vi "ShowRange.vi"(0 "File Info":T1={"FilePath"=path "/DATA/Labview Items", "Field (T)"=55.0, "Temperature (K)"=77.0, "X-Axis"=enum."nm", "Center nm"=55.0, "Current Grating Density"=enum."600", "CCD Parameters"={"Exposure Time (s)"=0.2, "Offset"=0.0, "BkgrdCrct"=FALSE, "Shutter"=FALSE, "Mode"=enum."Regular", "Repetition"=4, "dt or s"=0.0}, "Operation Mode"=enum."NML Data Acquisition", "Exp Index"=0, "Index_repetition"=0, "Index"=0, "Current Detector"=enum."CCD-1024x256"} {"CCD Parameters"."dt or s" format="%#.6f"; "CCD Parameters"."Repetition" min=1; "CCD Parameters"."Offset" format="%#.2f"; "CCD Parameters"."Exposure Time (s)" min=0.02 max=6000.0 format="%#.2f"; "Center nm" format="%.2f"; "Temperature (K)" format="%.2f"; "Field (T)" format="%.2f"}) -> ()   [LabVIEW 2020]
uses:
  Globals and TypeDefs/Type Definitions.llb/FileInfoParameter.ctt
  Globals and TypeDefs/Type Definitions.llb/Wavelength Unit.ctt
  Globals and TypeDefs/Type Definitions.llb/McPherson Grating Density.ctl
  Globals and TypeDefs/Type Definitions.llb/CCDParameter.ctt
  Globals and TypeDefs/Type Definitions.llb/OperationMode.ctt
  Globals and TypeDefs/Type Definitions.llb/ListOfDetectors.ctt
  X-Axis_Generator_x.vi
  X-Axis Converter.llb/X-Axis Converter.vi
panel:
  out "Old/Res/cm-1/500µ":dbl=118.16619973413901 caption="Old/Res/nm/10µ"
  out "Old/Res/cm-1/100µ":dbl=118.16619973413901 caption="Old/Res/nm/10µ" format="%.1f"
  out "New/Res/cm-1/500µ":dbl=25.810711007261716
  out "New/Res/cm-1/100µ":dbl=25.810711007261716 format="%.1f"
  out "Old/Res/cm-1/20µ":dbl=118.16619973413901 caption="Old/Res/nm/10µ" format="%.2f"
  out "New/Res/cm-1/20µ":dbl=25.810711007261716 format="%.2f"
  out "Old/Res/meV/500µ":dbl=118.16619973413901 caption="Old/Res/nm/10µ" format="%.1f"
  out "Old/Res/meV/100µ":dbl=118.16619973413901 caption="Old/Res/nm/10µ" format="%.2f"
  out "New/Res/meV/500µ":dbl=25.810711007261716 format="%.1f"
  out "New/Res/meV/100µ":dbl=25.810711007261716 format="%.2f"
  out "Old/Res/meV/20µ":dbl=118.16619973413901 caption="Old/Res/nm/10µ" format="%.3f"
  out "New/Res/meV/20µ":dbl=25.810711007261716 format="%.3f"
  out "Old/Res/nm/500µ":dbl=118.16619973413901 caption="Old/Res/nm/10µ" format="%.1f"
  out "Old/Res/nm/100µ":dbl=118.16619973413901 caption="Old/Res/nm/10µ" format="%.2f"
  out "New/Res/nm/500µ":dbl=25.810711007261716 format="%.1f"
  out "New/Res/nm/100µ":dbl=25.810711007261716 format="%.2f"
  out "Old/Res/nm/20µ":dbl=118.16619973413901 caption="Old/Res/nm/10µ" format="%.3f"
  out "New/Res/nm/20µ":dbl=25.810711007261716 format="%.3f"
  out "old cm-1 limit":dbl
  out "old meV limit":dbl
  out "old nm limit":dbl
  out "cm-1 limit":dbl
  out "meV limit":dbl
  out "nm limit":dbl
  out "Central WL output":dbl=619.92122 caption="Final Center Wavelength" format="%.2f"
  in  "Current Central WL":dbl=605.0 format="%.2f"
  in  "New Wavelength":dbl=619.92122 format="%.4f"
  in  "X-Axis":i32(ring)=1 items=["Point #", "nm", "eV", "meV", "cm-1"]
  out "Central cm-1 copy":dbl=16528.92561983471 caption="cm-1" format="%.2f"
  out "Central meV copy":dbl=2049.326347107438 caption="meV" format="%.3f"
  out "old Central Wavelength display":dbl=605.0 format="%.4f"
  out "old Current Grating Density":enum16{"150", "300", "600", "1200", "1800"}(ring)=enum."300" caption="old"
  in  "Current Grating Density":enum16{"150", "300", "600", "1200", "1800"}(ring)=enum."300"
  out "nm (delta) copy":dbl=118.16619973413901 format="%.4f"
  out "cm-1 (delta) copy":dbl=3261.1363066016183 format="%.2f"
  out "meV (delta) copy":dbl=404.32951820610924 format="%.2f"
  out "nm (Min) copy":dbl=545.7619367582628 format="%.4f"
  out "nm (Max) copy":dbl=663.9281364924018 format="%.4f"
  out "cm-1 (Max) copy":dbl=18323.00738926275 format="%.2f"
  out "cm-1 (Min) copy":dbl=15061.871082661133 format="%.2f"
  out "meV (Min) copy":dbl=1867.4346931794325 format="%.2f"
  out "meV (Max) copy":dbl=2271.764211385542 format="%.2f"
  out "Final Grating Density":enum16{"150", "300", "600", "1200", "1800"}(ring)=enum."1200" caption="Current"
  in  "New Grating Density":enum16{"150", "300", "600", "1200", "1800"}(ring)=enum."1200"
  in  "Return":bool
  in  "Central cm-1":dbl=16131.081946186647 caption="cm-1" format="%.2f"
  in  "Central meV":dbl=2000.0 caption="meV" format="%.3f"
  out "nm (delta)":dbl=25.810711007261716 format="%.4f"
  out "cm-1 (delta)":dbl=672.0827633332738 format="%.2f"
  out "meV (delta)":dbl=83.32767303932542 format="%.2f"
  out "nm (Min)":dbl=606.9391502209157 format="%.4f"
  out "nm (Max)":dbl=632.7498612281775 format="%.4f"
  out "cm-1 (Max)":dbl=16476.116257058333 format="%.2f"
  out "cm-1 (Min)":dbl=15804.033493725059 format="%.2f"
  out "meV (Max)":dbl=2042.7788113727688 format="%.2f"
  out "meV (Min)":dbl=1959.4511383334434 format="%.2f"
  in  "Central Wavelength":dbl=619.92122 caption="nm" format="%.4f"
  # "Parameters of Spectrometer System"
  # "Grating Density (grooves/mm)"
  # "New"
  # "Center Position"
  # "<"
  # ">"
  # ">"
  # "Mechnical Limit"
  # "Min"
  # "CCD Range"
  # "Max"
  # "D"
  # "20µ"
  # "100µ"
  # "Resolution"
  # "500µ"
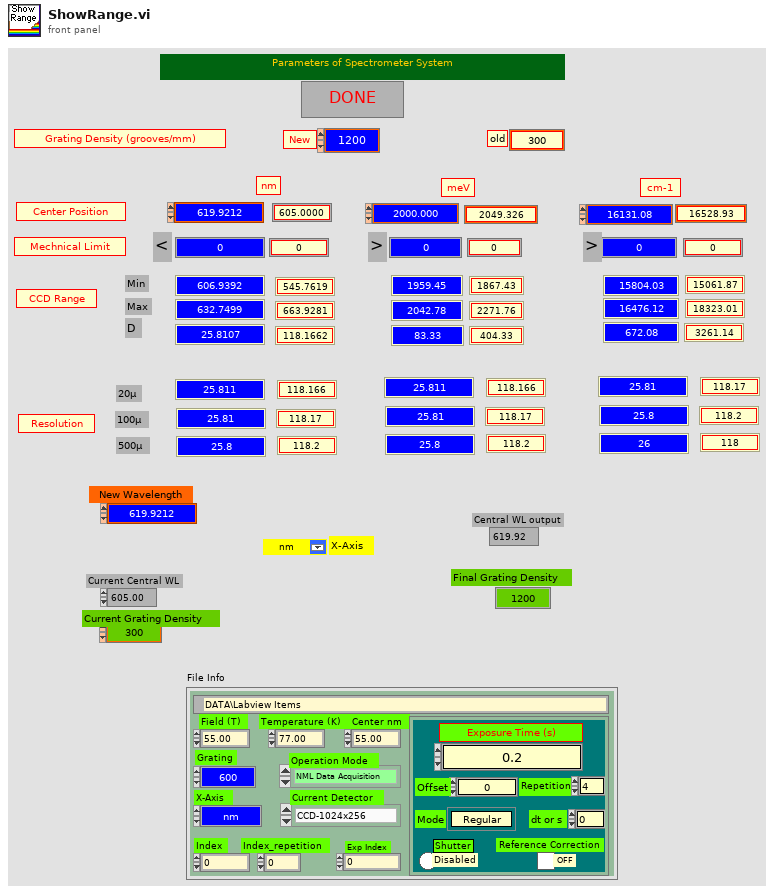
[diagram p1: front panel]
types:
  T1 = typedef "FileInfoParameter.ctt" = cluster{"FilePath":path, "Field (T)":dbl, "Temperature (K)":dbl, "X-Axis":T2, "Center nm":dbl, "Current Grating Density":T3, "CCD Parameters":T4, "Operation Mode":T5, "Exp Index":u32, "Index_repetition":u16, "Index":u16, "Current Detector":T6}
  T2 = typedef "Wavelength Unit.ctt" = enum8{"Point", "nm", "eV", "meV", "cm_1"}
  T3 = typedef "McPherson Grating Density.ctl" = enum8{"150", "300", "600", "1200", "1800"}
  T4 = typedef "CCDParameter.ctt" = cluster{"Exposure Time (s)":dbl, "Offset":dbl, "BkgrdCrct":bool, "Shutter":bool, "Mode":enum8{"Regular", "OverExp Cor", "SpikeRemove", "ForCalibration"}, "Repetition":u16, "dt or s":dbl}
  T5 = typedef "OperationMode.ctt" = enum16{"Standby", "CCD Single Shot", "CCD Sequence Shots", "CCD Custom Shots", "CCD Reference Shot", "Step Scanning ", "Time Scanning", "NML Data Acquisition"}
  T6 = typedef "ListOfDetectors.ctt" = enum8{"CCD-1024x256", "InGaAs PDA-1024x1", "CCD-1340x400", "Ge Single Channel", "Si Single Channel", "PMT Single Channel"}
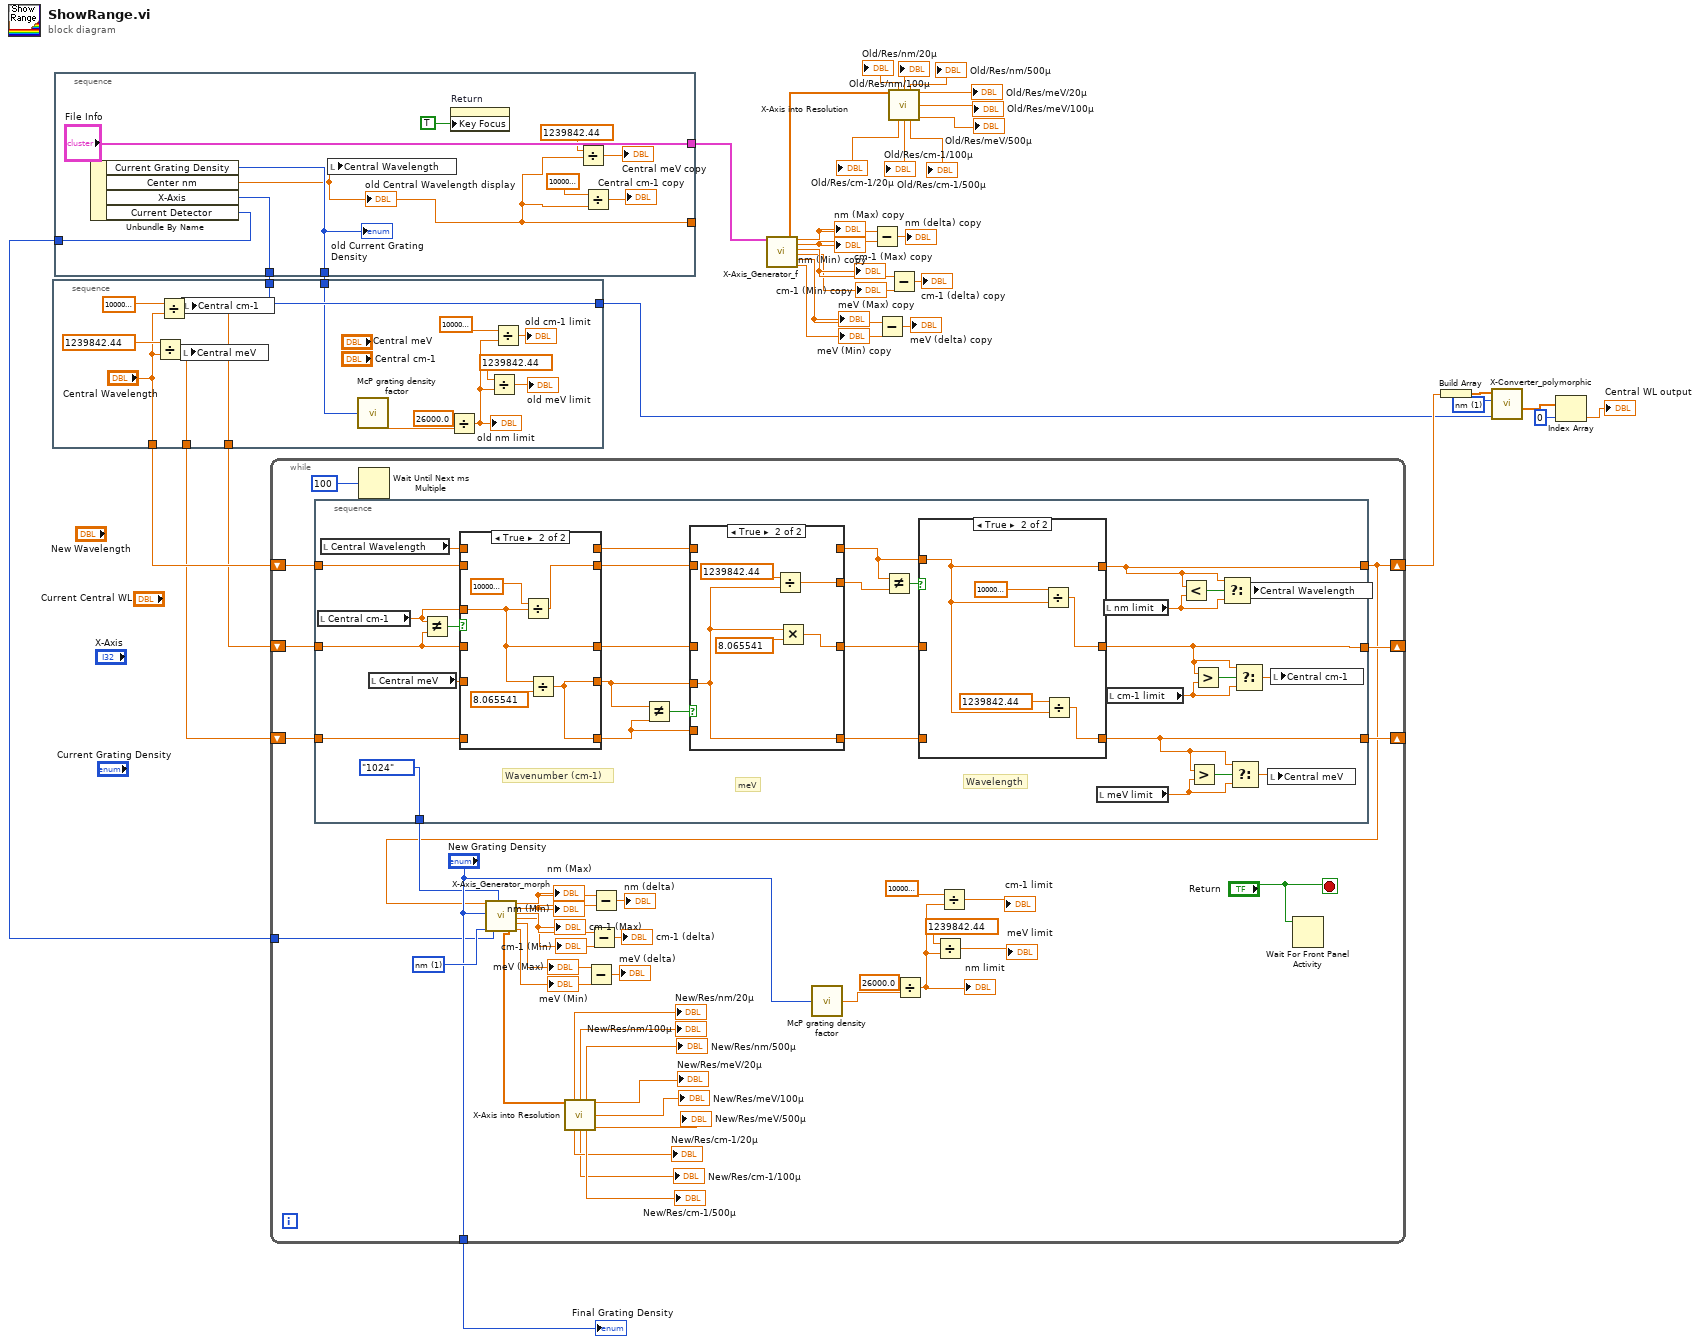
[diagram p0: block diagram]
diagram:
  w24 = 1 items=["Point #", "nm", "eV", "meV", "cm-1"] ("Old X-Axis Unit")
  n1 = stacked-sequence {
    tunnel: [w37] -> _
    tunnel: [w44] -> w23
    tunnel: [w42] -> w6
    tunnel: ["File Info"] -> w5
    tunnel: [w35] -> w1
    frame #0 {
      n2 = Unbundle By Name("File Info") -> ("Current Grating Density"=w42:T3, "Center nm"=w37:dbl, "X-Axis"=w44:T2, "Current Detector"=w35:T6)
      "old Central Wavelength display" <- w37
      "old Current Grating Density" <- w42
      n3 = local write "Central Wavelength"(w37) -> ()
      n4 = property on="Return" class="Bool"("Key Focus"=TRUE) -> ()  [unwired: 2 in, 2 out]
      n5 = Divide(x=1239842.44, y=w37) -> (x/y=→"Central meV copy":dbl)
      n6 = Divide(x=10000000.0, y=w37) -> (x/y=→"Central cm-1 copy":dbl)
    }
  }
  n7 = stacked-sequence {
    tunnel: w23 -> [w47]
    tunnel: ["Central Wavelength"] -> w21
    tunnel: [w48] -> w20
    tunnel: [w57] -> w19
    tunnel: [w47] -> w17
    tunnel: w6 -> [w45]
    frame #0 {
      n8 = Divide(x=1239842.44, y="Central Wavelength") -> (x/y=w48:dbl)
      n9 = Divide(x=10000000.0, y="Central Wavelength") -> (x/y=w57:dbl)
      n10 = local write "Central meV"(w48) -> ()
      n11 = local write "Central cm-1"(w57) -> ()
      n12 = call "McP grating density factor.vi"("Grating Density"=w45) -> ("GratingFactor"=w46:dbl)
      n13 = Divide(x=26000.0, y=w46) -> (x/y=w54:dbl)
      "old nm limit" <- w54
      n14 = Divide(x=1239842.44, y=w54) -> (x/y=→"old meV limit":dbl)
      n15 = Divide(x=10000000.0, y=w54) -> (x/y=→"old cm-1 limit":dbl)
    }
  }
  n16 = while {
    tunnel: ["New Grating Density"] -> w16
    shift-left: w20 -> [w80]
    shift-right: [w82] -> _
    shift-left: w19 -> [w81]
    shift-right: [w79] -> _
    shift-left: w21 -> [w78]
    shift-right: [w60] -> w18
    tunnel: w1 -> [w59]
    stop <- "Return" stop-if-true
    w77 = 1 items=["Point #", "nm", "eV", "meV", "cm-1"] ("X-Axis Unit")
    n17 = stacked-sequence {
      tunnel: [w103] -> w60
      tunnel: [w99] -> w82
      tunnel: w81 -> [w104]
      tunnel: w78 -> [w115]
      tunnel: w80 -> [w109]
      tunnel: [w101] -> w79
      tunnel: [enum16{"1024", "512", "3"}."1024" ("X-Axis Points")] -> w61
      frame #0 {
        # "Wavenumber (cm-1)"
        # "meV"
        # "Wavelength"
        n18 = local read "Central cm-1"() -> (w102:dbl)
        n19 = local read "Central Wavelength"() -> (w111:dbl)
        n20 = local read "Central meV"() -> (w110:dbl)
        n21 = Not Equal?(x=w102, y=w104) -> (x != y?=w125:bool)
        n22 = case shown="True" w125 {
          tunnel: w102 -> [_ w134]
          tunnel: [w132 w135] -> w114
          tunnel: w115 -> [w132 _]
          tunnel: [w131 w135] -> w112
          tunnel: w111 -> [w131 _]
          tunnel: [w130 w133] -> w100
          tunnel: w110 -> [w130 _]
          tunnel: w109 -> [w129 _]
          tunnel: [w129 w133] -> w106
          tunnel: [w128 w134] -> w107
          tunnel: w104 -> [w128 _]
          frame False {
          }
          frame True {
            n23 = Divide(x=10000000.0, y=w134) -> (x/y=w135:dbl)
            n24 = Divide(x=w134, y=8.065541) -> (x/y=w133:dbl)
          }
        }
        n25 = Not Equal?(x=w100, y=w106) -> (x != y?=w126:bool)
        n26 = case shown="True" w126 {
          tunnel: [w141 w144] -> w113
          tunnel: w114 -> [w141 _]
          tunnel: [w140 w144] -> w98
          tunnel: w112 -> [w140 _]
          tunnel: w100 -> [_ w142]
          tunnel: [w139 w143] -> w108
          tunnel: w107 -> [w139 _]
          tunnel: [w138 w142] -> w105
          tunnel: w106 -> [w138 _]
          frame False {
          }
          frame True {
            n27 = Divide(x=1239842.44, y=w142) -> (x/y=w144:dbl)
            n28 = Multiply(x=w142, y=8.065541) -> (x*y=w143:dbl)
          }
        }
        n29 = Not Equal?(x=w98, y=w113) -> (x != y?=w127:bool)
        n30 = case shown="True" w127 {
          tunnel: w98 -> [w149 w152]
          tunnel: [w149 w152] -> w103
          tunnel: [w147 w150] -> w99
          tunnel: w108 -> [w148 _]
          tunnel: [w148 w151] -> w101
          tunnel: w105 -> [w147 _]
          frame False {
          }
          frame True {
            n31 = Divide(x=10000000.0, y=w152) -> (x/y=w151:dbl)
            n32 = Divide(x=1239842.44, y=w152) -> (x/y=w150:dbl)
          }
        }
        n33 = local read "meV limit"() -> (w119:dbl)
        n34 = local read "nm limit"() -> (w117:dbl)
        n35 = local read "cm-1 limit"() -> (w123:dbl)
        n36 = Less?(x=w103, y=w117) -> (x < y?=w120:bool)
        n37 = Greater?(x=w99, y=w119) -> (0:w121:bool)
        n38 = Greater?(x=w101, y=w123) -> (0:w124:bool)
        n39 = Select(t=w103, s=w120, f=w117) -> (s? t:f=w116:dbl)
        n40 = Select(t=w99, s=w121, f=w119) -> (s? t:f=w118:dbl)
        n41 = Select(t=w101, s=w124, f=w123) -> (s? t:f=w122:dbl)
        n42 = local write "Central Wavelength"(w116) -> ()
        n43 = local write "Central meV"(w118) -> ()
        n44 = local write "Central cm-1"(w122) -> ()
      }
    }
    n45 = Wait Until Next ms Multiple(millisecond multiple=u32 100) -> ()  [unwired: 1 out]
    n46 = call-poly "X-Axis_Generator_morph.vi"("Central Wavelength"=w60, "Current Grating Density"="New Grating Density", "X-Axis Unit"=w77, "Current Detector"=w59, "X-Axis Points"=w61) -> ("X-axis"=w76:dbl[], "nm (Max)"=w95:dbl, "nm (Min)"=w94:dbl, "cm-1 (Max)"=w63:dbl, "cm-1 (Min)"=w62:dbl, "meV (Max)"=w90:dbl, "meV (Min)"=w89:dbl)  [unwired: 7 in, 1 out]
    "nm (Min)" <- w94
    "nm (Max)" <- w95
    "cm-1 (Max)" <- w63
    "cm-1 (Min)" <- w62
    "meV (Min)" <- w89
    "meV (Max)" <- w90
    n47 = call "X-Axis into Resolution.vi"("X-axis (nm)"=w76) -> ("Res/nm/20µ"=→"New/Res/nm/20µ":dbl, "Res/nm/100µ"=→"New/Res/nm/100µ":dbl, "Res/nm/500µ"=→"New/Res/nm/500µ":dbl, "Res/meV/20µ"=→"New/Res/meV/20µ":dbl, "Res/meV/100µ"=→"New/Res/meV/100µ":dbl, "Res/cm-1/20µ"=→"New/Res/cm-1/20µ":dbl, "Res/cm-1/100µ"=→"New/Res/cm-1/100µ":dbl, "Res/cm-1/500µ"=→"New/Res/cm-1/500µ":dbl, "Res/meV/500"=→"New/Res/meV/500µ":dbl)  [unwired: 6 in]
    n48 = Subtract(x=w90, y=w89) -> (x-y=→"meV (delta)":dbl)
    n49 = Subtract(x=w63, y=w62) -> (x-y=→"cm-1 (delta)":dbl)
    n50 = Subtract(x=w95, y=w94) -> (x-y=→"nm (delta)":dbl)
    n51 = call "McP grating density factor.vi"("Grating Density"="New Grating Density") -> ("GratingFactor"=w65:dbl)
    n52 = Divide(x=26000.0, y=w65) -> (x/y=w83:dbl)
    "nm limit" <- w83
    n53 = Divide(x=1239842.44, y=w83) -> (x/y=→"meV limit":dbl)
    n54 = Divide(x=10000000.0, y=w83) -> (x/y=→"cm-1 limit":dbl)
    n55 = Wait For Front Panel Activity(3:"Return") -> ()  [unwired: 2 in, 1 out]
  }
  "Final Grating Density" <- w16
  n56 = call-poly "X-Axis_Generator_f.vi"("File Info In"=w5) -> ("X-axis  (nm)"=w4:dbl[], "nm (Max)"=w34:dbl, "nm (Min)"=w33:dbl, "cm-1 (Max)"=w3:dbl, "cm-1 (Min)"=w2:dbl, "meV (Max)"=w29:dbl, "meV (Min)"=w28:dbl)  [unwired: 11 in, 1 out]
  "nm (Min) copy" <- w33
  "nm (Max) copy" <- w34
  "cm-1 (Max) copy" <- w3
  "cm-1 (Min) copy" <- w2
  "meV (Min) copy" <- w28
  "meV (Max) copy" <- w29
  n57 = Subtract(x=w34, y=w33) -> (x-y=→"nm (delta) copy":dbl)
  n58 = Subtract(x=w29, y=w28) -> (x-y=→"meV (delta) copy":dbl)
  n59 = call "X-Axis into Resolution.vi"("X-axis (nm)"=w4) -> ("Res/nm/20µ"=→"Old/Res/nm/20µ":dbl, "Res/nm/100µ"=→"Old/Res/nm/100µ":dbl, "Res/nm/500µ"=→"Old/Res/nm/500µ":dbl, "Res/meV/20µ"=→"Old/Res/meV/20µ":dbl, "Res/meV/100µ"=→"Old/Res/meV/100µ":dbl, "Res/cm-1/20µ"=→"Old/Res/cm-1/20µ":dbl, "Res/cm-1/100µ"=→"Old/Res/cm-1/100µ":dbl, "Res/cm-1/500µ"=→"Old/Res/cm-1/500µ":dbl, "Res/meV/500"=→"Old/Res/meV/500µ":dbl)  [unwired: 6 in]
  n60 = Subtract(x=w3, y=w2) -> (x-y=→"cm-1 (delta) copy":dbl)
  n61 = Build Array(w18) -> (w27:dbl[])
  n62 = call-poly "X-Converter_polymorphic.vi"("X-Axis Unit"=w17, "Old X-Axis Unit"=w24, "X-Axis input"=w27) -> ("X-Axis Output"=w26:dbl[])  [unwired: 2 in, 3 out]
  n63 = Index Array(array=w26, index=0) -> (element=→"Central WL output":dbl)
